vi "Move Error Wires to Background.vi"(6 "Variant in":variant, 7 "Shift Pressed?":bool, 8 "error in (no error)":errorcluster, 10 "QD Combo Box Ref":refnum<vi>, 11 "QD Launch VI Ref":refnum<vi>) -> (0 "error out":errorcluster, 4 "Variant out":variant)   [LabVIEW 2019]
doc: "If items are selected when this shortcut executes then the selection will be forced to the background. However, if no items are selected. This shortcut will send all error wires to the background\nThis shortcut will only execute on the block diagram.\n\nDefault Shortcut - [e]"
uses:
  <vilib>/Utility/traverseref.llb/TRef TravTarget.ctl
  <vilib>/addons/analyzer/_analyzerutils.llb/VIAnUtil Check Type If ErrClust.vi
  <vilib>/Utility/traverseref.llb/VI Scripting - Traverse.lvlib
  <vilib>/Utility/Data Type/NI_Data Type.lvlib
panel:
  in  "Undo Name":string="Quick Drop Keyboard Shortcut"
  # "Do not change the connector pane of this VI.\n\nSee the block diagram for directions on how to use this template."
  # "Specify the name of the Undo transaction"
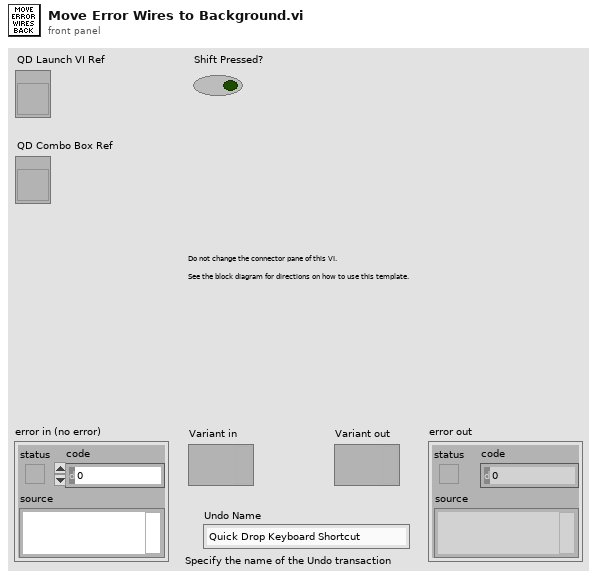
[diagram p1: front panel]
types:
  T1 = typedef "TRef TravTarget.ctl" = enum16{"FP", "BD", "Other"}
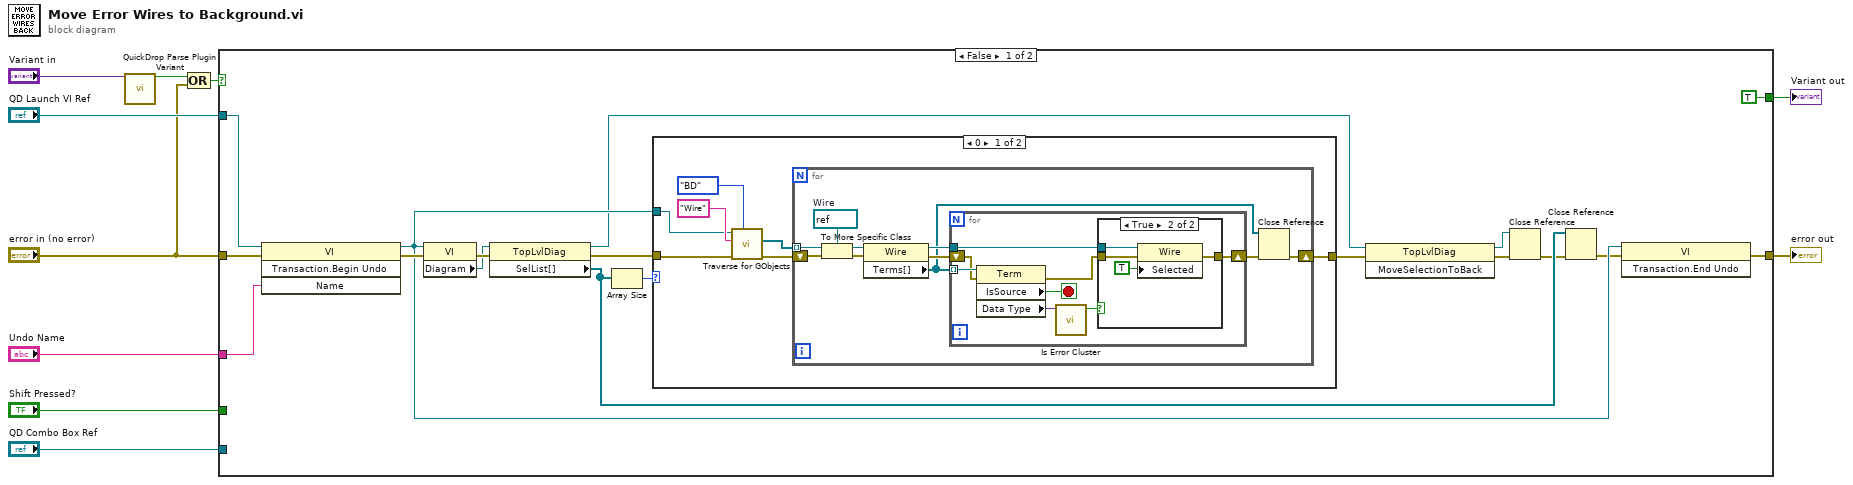
[diagram p0: block diagram]
diagram:
  n1 = call <vilib>:"QuickDrop Parse Plugin Variant.vi"("QDKS Variant in"="Variant in") -> ("QD Launch VI Panel?"=w3:bool)  [unwired: 12 in, 2 out]
  n2 = Compound Arithmetic op=OR(w3, "error in (no error)") -> (w1:bool)
  n3 = case shown="False" w1 {
    tunnel: [w23 w60] -> w10
    tunnel: "QD Launch VI Ref" -> [w27 _]
    tunnel: "Shift Pressed?" -> [_ _]
    tunnel: "QD Combo Box Ref" -> [_ _]
    tunnel: "Undo Name" -> [w26 _]
    tunnel: [TRUE _] -> w5
    tunnel: "error in (no error)" -> [w28 w60]
    frame False {
      n4 = invoke class="VI" method="Transaction.Begin Undo"(reference=w27, error in=w28, "Name"=w26) -> (reference out=w19:refnum<vi>, error out=w24:errorcluster)  [unwired: 1 in, 2 out]
      n5 = property class="VI"(reference=w19, error in=w24) -> (error out=w22:errorcluster, "Diagram"=w21:refnum<vi>)  [unwired: 1 out]
      n6 = property class="TopLvlDiag"(reference=w21, error in=w22) -> (reference out=w17:refnum<vi>, error out=w18:errorcluster, "SelList[]"=w15:refnum<vi>[])
      n7 = Array Size(array=w15) -> (size(s)=w20:i32)
      n8 = case shown="0" w20 {
        tunnel: w19 -> [w31 _]
        tunnel: w18 -> [w30 w59]
        tunnel: [w29 w59] -> w16
        frame 0 {
          n9 = call <vilib>:"Traverse for GObjects.vi"("Traverse Target"=TRef_TravTarget."BD", "error in (no error)"=w30, "Class Name"="Wire", "VI Refnum"=w31) -> ("error out"=w32:errorcluster, "References"=w33:refnum<vi>[])  [unwired: 4 in, 2 out]
          n10 = for {
            tunnel: w33 -> [w45] mode=indexing
            shift-right: [w37] -> w29
            shift-left: w32 -> [w40]
            w39 = refnum<vi> refnum  # Wire
            n11 = To More Specific Class(target class=w39, reference=w45, error in=w40) -> (specific class reference=w44:refnum<vi>, error out=w42:errorcluster)
            n12 = property class="Wire"(reference=w44, error in=w42) -> (reference out=w43:refnum<vi>, error out=w41:errorcluster, "Terms[]"=w36:refnum<vi>[])
            n13 = for {
              tunnel: w36 -> [w53] mode=indexing
              tunnel: w43 -> [w49]
              shift-right: [w47] -> w38
              shift-left: w41 -> [w48]
              stop <- w52 stop-if-true
              n14 = property class="Term"(reference=w53, error in=w48) -> (error out=w46:errorcluster, "IsSource"=w52:bool, "Data Type"=w51:variant)  [unwired: 1 out]
              n15 = call <vilib>:"Is Error Cluster.vi"("variant"=w51) -> ("is error cluster?"=w50:bool)  [unwired: 9 in, 1 out]
              n16 = case shown="True" w50 {
                tunnel: w49 -> [_ w58]
                tunnel: w46 -> [w54 w56]
                tunnel: [w54 w55] -> w47
                frame False {
                }
                frame True {
                  n17 = property class="Wire"(reference=w58, error in=w56, "Selected"=TRUE) -> (error out=w55:errorcluster)  [unwired: 1 out]
                }
              }
            }
            n18 = Close Reference(reference=w36, error in (no error)=w38) -> (error out=w37:errorcluster)
          }
        }
        frame Default {
        }
      }
      n19 = invoke class="TopLvlDiag" method="MoveSelectionToBack"(reference=w17, error in=w16) -> (reference out=w14:refnum<vi>, error out=w13:errorcluster)  [unwired: 1 in, 1 out]
      n20 = Close Reference(reference=w14, error in (no error)=w13) -> (error out=w12:errorcluster)
      n21 = Close Reference(reference=w15, error in (no error)=w12) -> (error out=w11:errorcluster)
      n22 = invoke class="VI" method="Transaction.End Undo"(reference=w19, error in=w11) -> (error out=w23:errorcluster)  [unwired: 1 in, 2 out]
    }
    frame True {
    }
  }
  "error out" <- w10
  "Variant out" <- w5
